vi "queryTelemetry.vi"   [LabVIEW 2015]
uses:
  DataTypes/QueryTelemetryLoop.ctl
  DataTypes/QueryTelemetryStates.ctl
  <vilib>/rvi/Emulation/niFpgaGetClockAttributes.vi
  <vilib>/rvi/Emulation/niFpgaSctlEmulationGetInTimedLoop.vi
  <vilib>/rvi/Emulation/niFpgaEmulationReportErrorSimple.vi
  <vilib>/rvi/Emulation/niFpgaEmulationIsFPGAContextNoSignature.vi
  <vilib>/rvi/DataTransferAndStorage/Container/Common/niFpgaContainerGetUniqueNameForEmu.vi
  <vilib>/rvi/Memory/Memory_Emulation/niFpgaMemoryEmulationCacheClearOnFirstRun.vi
  <vilib>/rvi/Memory/Memory_Emulation/nirvimemoryEmulationManagerCache_MakeExclusive.vi
  <vilib>/rvi/Memory/Memory_Emulation/niFpgaMemoryEmulationValidateCache.vi
  <vilib>/rvi/Memory/Memory_Emulation/nirvimemoryEmulationManagerCache_InsertValue.vi
  <vilib>/Utility/error.llb/Clear Errors.vi
  <vilib>/rvi/Memory/Memory_Emulation/nirvimemoryEmulationManagerCache_ReleaseExclusive.vi
  <vilib>/rvi/Memory/Memory_Emulation/nirvimemoryEmulationManagerCache_GetValue.vi
  <vilib>/rvi/Memory/Memory_Emulation/nirvimemoryEmulationManagerCache_SetValue.vi
  <vilib>/rvi/Emulation/niFpgaProcessEmulError.vi
  <vilib>/rvi/Memory/Memory_Emulation/nirvimemoryFastEmulation.vi
  <vilib>/rvi/Memory/Memory_Emulation/nirvimemoryEmulation.vi
  <vilib>/rvi/errors/nirviReportUnexpectedCaseInternalError (U32).vi
  <vilib>/rvi/interface/RandomDataEmulation/niFpgaRandomDataHandleErrors.vi
  <vilib>/rvi/Emulation/niFpgaCriticalErrorInLSC.vi
  <vilib>/rvi/DataTransferAndStorage/Container/XNode/niFpgaContainer.xnode
  <vilib>/rvi/DataTransferAndStorage/Register/Emulation/niFpgaRegisterEmulation.vi
  <vilib>/rvi/interface/RandomDataEmulation/nirviRandomDataFpgaReadWriteTemplate.vi
types:
  T1 = typedef "QueryTelemetryLoop.ctl" = cluster{"State":T2, "Instruction Data":u32, "Telemetry Offset":u32}
  T2 = typedef "QueryTelemetryStates.ctl" = enum16{"Try Read Instruction", "Send Telemetry", "Send All Telemetry"}
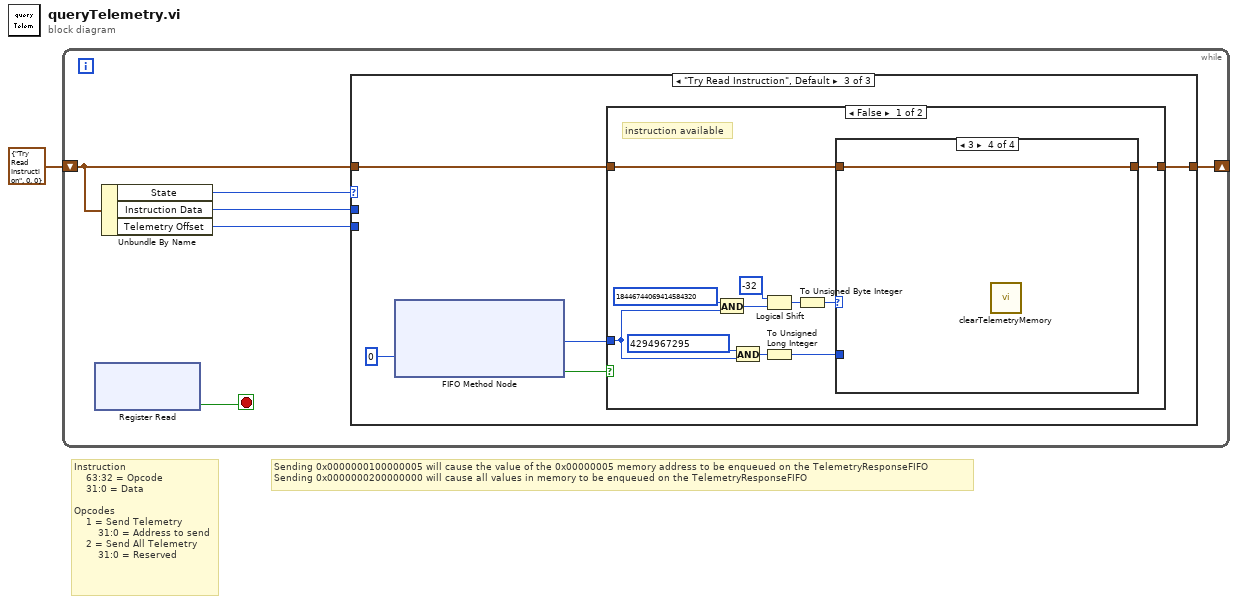
[diagram p0: block diagram]
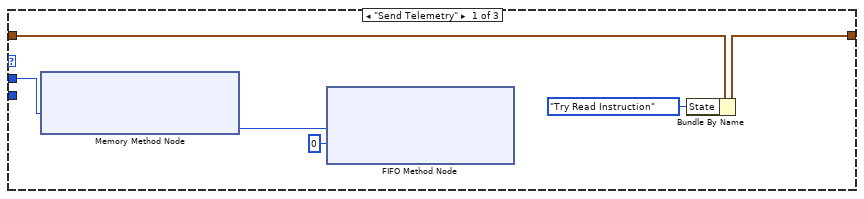
[diagram p2: hidden frame]
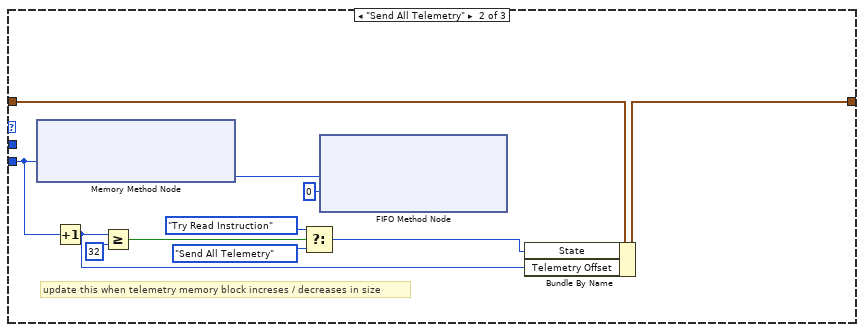
[diagram p3: hidden frame]
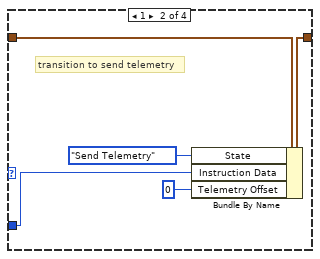
[diagram p5: hidden frame]
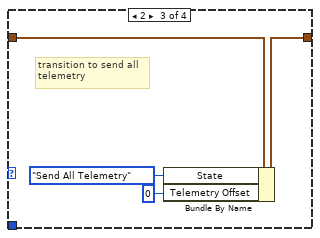
[diagram p6: hidden frame]
diagram:
  # "Sending 0x0000000100000005 will cause the value of the 0x00000005 memory address to be enqueued on the TelemetryResponseFIFO\nSending 0x0000000200000000 will cause all values in memory to be enqueued on the TelemetryResponseFIFO"
  # "Instruction\n    63:32 = Opcode\n    31:0 = Data\n\nOpcodes\n    1 = Send Telemetry\n        31:0 = Address to send\n    2 = Send All Telemetry\n        31:0 = Reserved"
  n1 = while {
    shift-right: [w3] -> _
    shift-left: T1 {"State"=enum."Try Read Instruction", "Instruction Data"=0, "Telemetry Offset"=0} ("Command Telemetry Loop") -> [w6]
    stop <- w4 stop-if-true
    n2 = xnode ("Register Read")() -> ("Data"=w4:bool)  [unwired: 1 in, 1 out]
    n3 = Unbundle By Name(w6) -> ("State"=w7:T2, "Instruction Data"=w5:u32, "Telemetry Offset"=w2:u32)
    n4 = case shown="\"Try Read Instruction\", Default" w7 {
      tunnel: w6 -> [w13 w24 w28]
      tunnel: w5 -> [w11 _ _]
      tunnel: [w12 w23 w27] -> w3
      tunnel: w2 -> [_ w20 _]
      frame "Send Telemetry" {
        n5 = xnode ("Memory Method Node")("Address"=w11) -> ("Data"=w9:u32)  [unwired: 1 in, 1 out]
        n6 = xnode ("FIFO Method Node")("Element"=w9, "Timeout"=0) -> ()  [unwired: 1 in, 2 out]
        n7 = Bundle By Name(cluster=w13, "State"=QueryTelemetryStates."Try Read Instruction" ("f")) -> (w12:T1)
      }
      frame "Send All Telemetry" {
        # "update this when telemetry memory block increses / decreases in size"
        n8 = xnode ("Memory Method Node")("Address"=w20) -> ("Data"=w22:u32)  [unwired: 1 in, 1 out]
        n9 = Increment(x=w20) -> (x+1=w14:u32)
        n10 = Greater Or Equal?(x=w14, y=u32 32) -> (x >= y?=w18:bool)
        n11 = Select(t=QueryTelemetryStates."Try Read Instruction" ("f"), s=w18, f=QueryTelemetryStates."Send All Telemetry") -> (s? t:f=w15:T2)
        n12 = xnode ("FIFO Method Node")("Element"=w22, "Timeout"=0) -> ()  [unwired: 1 in, 2 out]
        n13 = Bundle By Name(cluster=w24, "State"=w15, "Telemetry Offset"=w14) -> (w23:T1)
      }
      frame "Try Read Instruction", Default {
        n14 = xnode ("FIFO Method Node")("Timeout"=0) -> ("Element"=w29:u64, "Timed Out?"=w25:bool)  [unwired: 1 in, 1 out]
        n15 = case shown="False" w25 {
          tunnel: w29 -> [w30 _]
          tunnel: w28 -> [w40 w52]
          tunnel: [w39 w52] -> w27
          frame False {
            # "instruction available"
            n16 = And(x=u64 18446744069414584320, y=w30) -> (x .and. y?=w36:u64)
            n17 = And(x=u64 4294967295, y=w30) -> (x .and. y?=w32:u64)
            n18 = Logical Shift(y=i16 -32, x=w36) -> (x << y=w34:u64)
            n19 = To Unsigned Long Integer(number=w32) -> (unsigned 32bit integer=w31:u32)
            n20 = To Unsigned Byte Integer(number=w34) -> (unsigned 8bit integer=w33:u8)
            n21 = case shown="3" w33 {
              tunnel: w40 -> [w41 w46 w50 w51]
              tunnel: [w41 w45 w49 w51] -> w39
              tunnel: w31 -> [_ w42 _ _]
              frame 0, Default {
                # "nop"
              }
              frame 1 {
                # "transition to send telemetry"
                n22 = Bundle By Name(cluster=w46, "State"=QueryTelemetryStates."Send Telemetry", "Instruction Data"=w42, "Telemetry Offset"=u32 0) -> (w45:T1)
              }
              frame 2 {
                # "transition to send all \ntelemetry"
                n23 = Bundle By Name(cluster=w50, "State"=QueryTelemetryStates."Send All Telemetry", "Telemetry Offset"=u32 0) -> (w49:T1)
              }
              frame 3 {
                n24 = call "clearTelemetryMemory.vi"() -> ()  [unwired: 12 in]
              }
            }
          }
          frame True {
            # "no instruction available"
          }
        }
      }
    }
  }
